vi "Format CSV Data.vi"(11 "String Array Row":string[](array[string])) -> (3 "Formatted Row":string)   [LabVIEW 2022 SP3, in "CSV Export.lvlib" / "CSV Export.lvclass"]
uses:
  CSV Export.lvclass
panel:
  # "IVB Data Logging - Format Row String Data.vi\n\nThis VI formats an array of strings into a single string that is either tab delimeted or commas separated depending on the File Type.  A return carriage is added to the end of the resulting string."
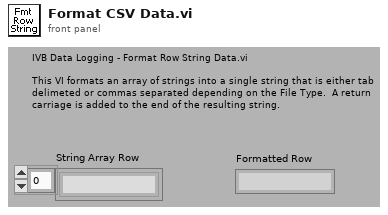
[diagram p1: front panel]
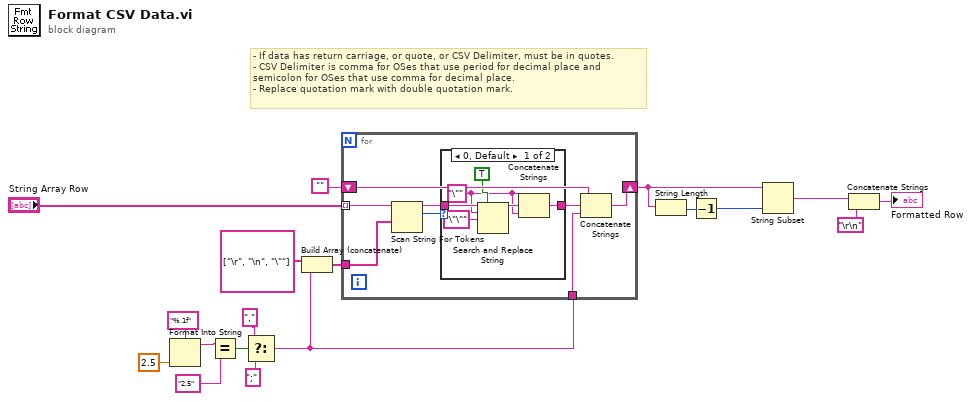
[diagram p0: block diagram]
diagram:
  # "- If data has return carriage, or quote, or CSV Delimiter, must be in quotes.\n- CSV Delimiter is comma for OSes that use period for decimal place and semicolon for OSes that use comma for decimal place.\n- Replace quotation mark with double quotation mark."
  n1 = Format Into String(format string="%.1f", 2.5 ("input 1")) -> (resulting string=w12:string)  [unwired: 2 in, 1 out]
  n2 = Equal?(x=w12, y="2.5") -> (x = y?=w9:bool)
  n3 = Select(t=",", s=w9, f=";") -> (s? t:f=w5:string)
  n4 = Build Array (concatenate)(string[] ["\r", "\n", "\""] ("operators (none)"), w5) -> (w6:string[])
  n5 = for {
    tunnel: "String Array Row" -> [w23] mode=indexing
    tunnel: w6 -> [w25]
    shift-right: [w20] -> w3
    shift-left: "" -> [w19]
    tunnel: w5 -> [w21]
    n6 = Scan String For Tokens(7:w25, 9:w23) -> (2:w24:i32)  [unwired: 4 in, 3 out]
    n7 = case shown="0, Default" w24 {
      tunnel: w23 -> [w31 w32]
      tunnel: [w27 w32] -> w22
      frame 0, Default {
        w26 = "\"" ("search string")
        n8 = Search and Replace String(replace all?=TRUE ("replace all? (F)"), input string=w31, search string=w26, replace string="\"\"" ("replace string (\"\")")) -> (result string=w28:string)  [unwired: 4 in, 3 out]
        n9 = Concatenate Strings(w26, w28, w26) -> (w27:string)
      }
      frame -1 {
        # "No special chars"
      }
    }
    n10 = Concatenate Strings(w19, w22, w21) -> (w20:string)
  }
  n11 = String Length(string=w3) -> (length=w2:i32)
  n12 = Decrement(x=w2) -> (x-1=w1:i32)
  n13 = String Subset(string=w3, length (rest)=w1) -> (substring=w16:string)  [unwired: 1 in]
  n14 = Concatenate Strings(w16, "\r\n") -> (→"Formatted Row":string)
